vi "makeClampWvfrm_ItoV.vi"(11 "Current in (pA)":dbl) -> (3 "cmd voltage (V)":dbl)   [LabVIEW 2019]
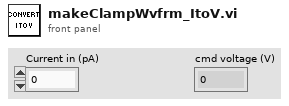
[diagram p1: front panel]
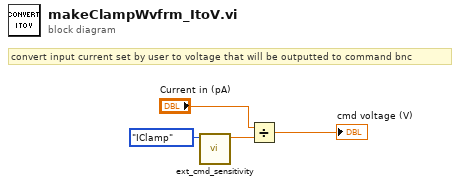
[diagram p0: block diagram]
diagram:
  # "convert input current set by user to voltage that will be outputted to command bnc"
  n1 = call "ext_cmd_sensitivity.vi"("which clamp"=enum16{"VClamp", "IClamp"}."IClamp") -> ("division factor"=w3:dbl)  [unwired: 10 in]
  n2 = Divide(x="Current in (pA)", y=w3) -> (x/y=→"cmd voltage (V)":dbl)
